vi "MeasureIdd.vi"(8 "error in (no error)":errorcluster, 9 "Deep Sleep Time":u32, 10 "channel name":string="0", 11 "instrument handle":refnum<k15>) -> (0 "error out":errorcluster, 2 "Idd Average":dbl format="%0.2f", 3 "instrument handle out":refnum<k15>)   [LabVIEW 2018]
uses:
  <instrlib>/niDCPower/nidcpower.llb/niDCPower Measurement Type.ctl
  <vilib>/Analysis/baseanly.llb/Mean (DBL).vi
  <vilib>/Analysis/NI_AALBase.lvlib
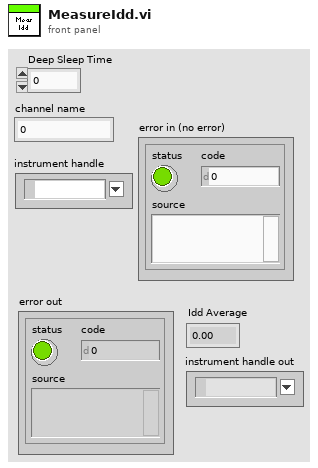
[diagram p1: front panel]
types:
  T1 = typedef "niDCPower Measurement Type.ctl" = i32
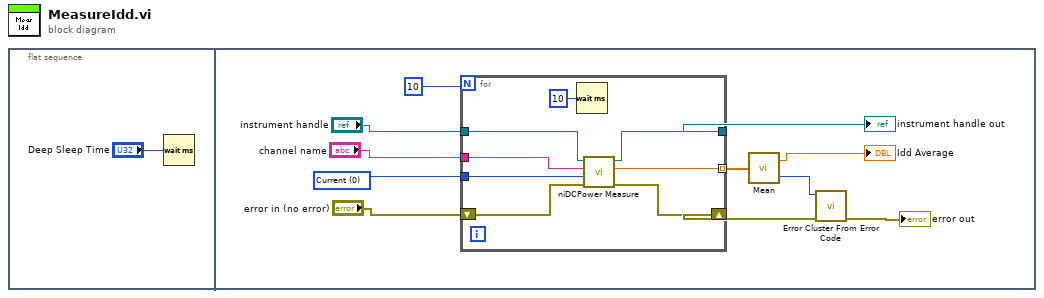
[diagram p0: block diagram]
diagram:
  n1 = flat-sequence {
    frame #0 {
      n2 = Wait (ms)(milliseconds to wait="Deep Sleep Time") -> ()  [unwired: 1 out]
    }
    frame #1 {
      w8 = T1 0 items=["Current", "Voltage"] ("measurement type")
      n3 = for {
        N: 10 -> [_]
        tunnel: w8 -> [w20]
        tunnel: [w17] -> w12 mode=indexing
        tunnel: "channel name" -> [w15]
        shift-right: [w18] -> w4
        shift-left: "error in (no error)" -> [w19]
        tunnel: "instrument handle" -> [w14]
        tunnel: [w16] -> w2
        n4 = Wait (ms)(milliseconds to wait=u32 10) -> ()  [unwired: 1 out]
        n5 = call <instrlib>:"niDCPower Measure.vi"("error in (no error)"=w19, "measurement type"=w20, "channel name"=w15, "instrument handle"=w14) -> ("error out"=w18:errorcluster, "measurement"=w17:dbl, "instrument handle out"=w16:refnum<k15>)  [unwired: 5 in]
      }
      "instrument handle out" <- w2
      n6 = call-poly <vilib>:"Mean.vi"("X"=w12) -> ("mean"=→"Idd Average":dbl, "error"=w3:i32)
      n7 = call <vilib>:"Error Cluster From Error Code.vi"("error in (no error)"=w4, "error code (0)"=w3) -> ("error out"=→"error out":errorcluster)  [unwired: 7 in]
    }
  }
